vi "Recognize correct target fixed.vi"(9 "# rectangles":i32, 10 "Rectangles (Calibrated)":T2(array[cluster]), 11 "Image":T1) -> (3 "Image Out":T1)   [LabVIEW 2018]
uses:
  <vilib>/vision/Image Controls.llb/IMAQ Image.ctl
  Dashboard globals.vi
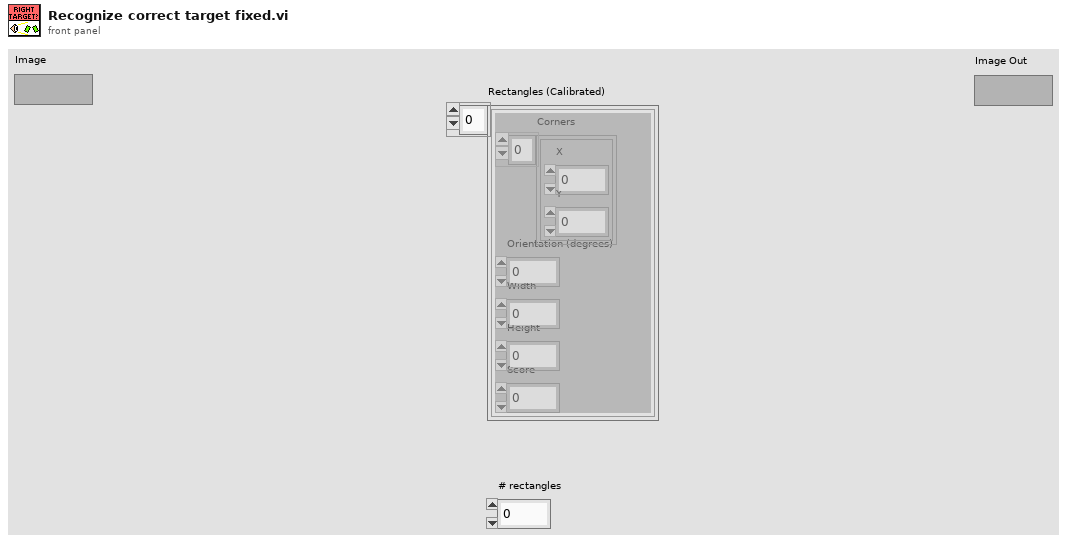
[diagram p1: front panel]
types:
  T1 = typedef "IMAQ Image.ctl" = refnum<image>
  T2 = cluster{"Corners":cluster{"X":sgl, "Y":sgl}[], "Orientation (degrees)":dbl, "Width":dbl, "Height":dbl, "Score":dbl}[]
  T3 = enum32{"Ship Left", "Ship Center", "Ship Right", "Rocket or Loading Station"}
  T4 = cluster{"Corners":cluster{"X":sgl, "Y":sgl}[], "Orientation (degrees)":dbl, "Width":dbl, "Height":dbl, "Score":dbl}
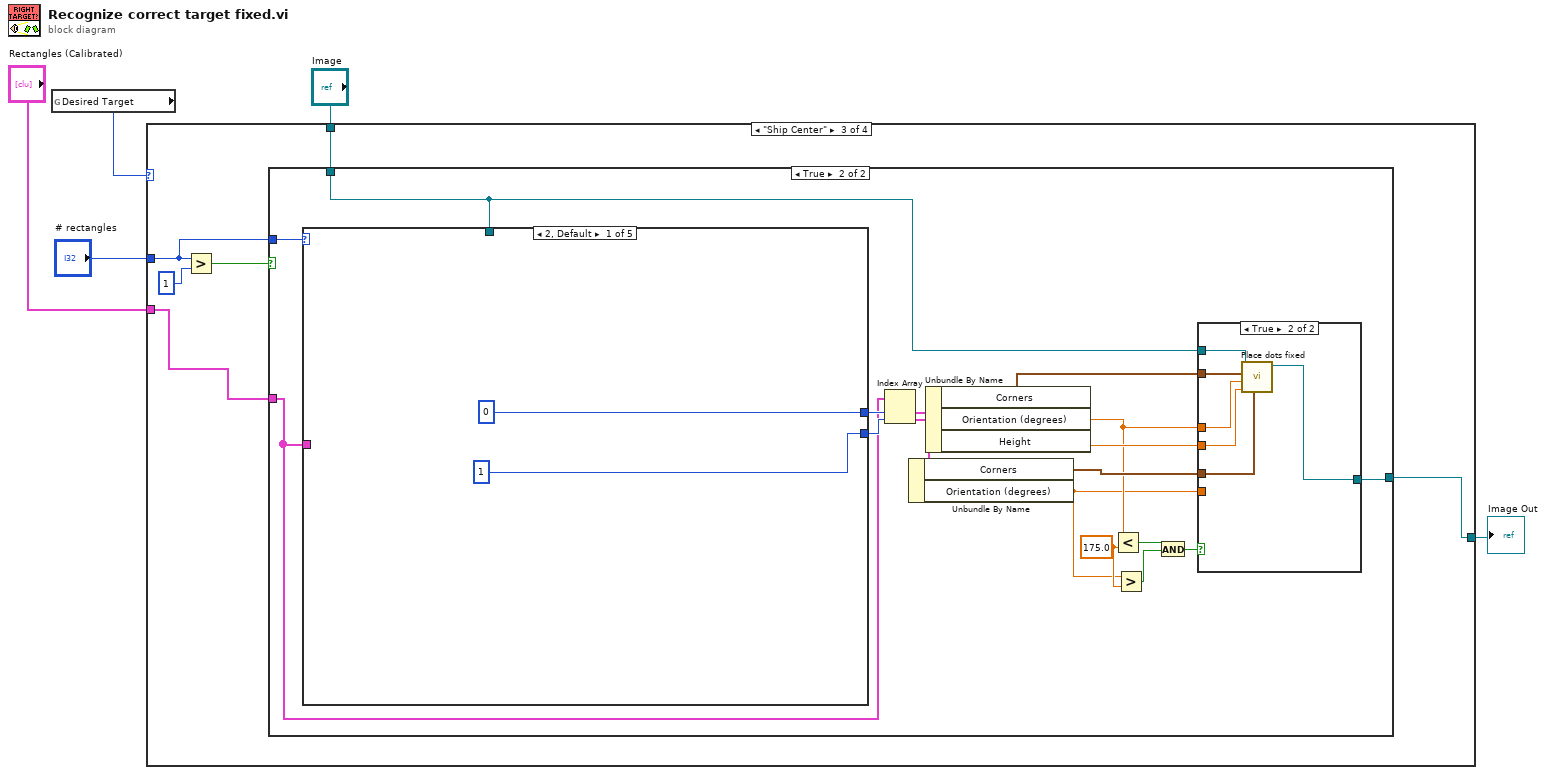
[diagram p0: block diagram]
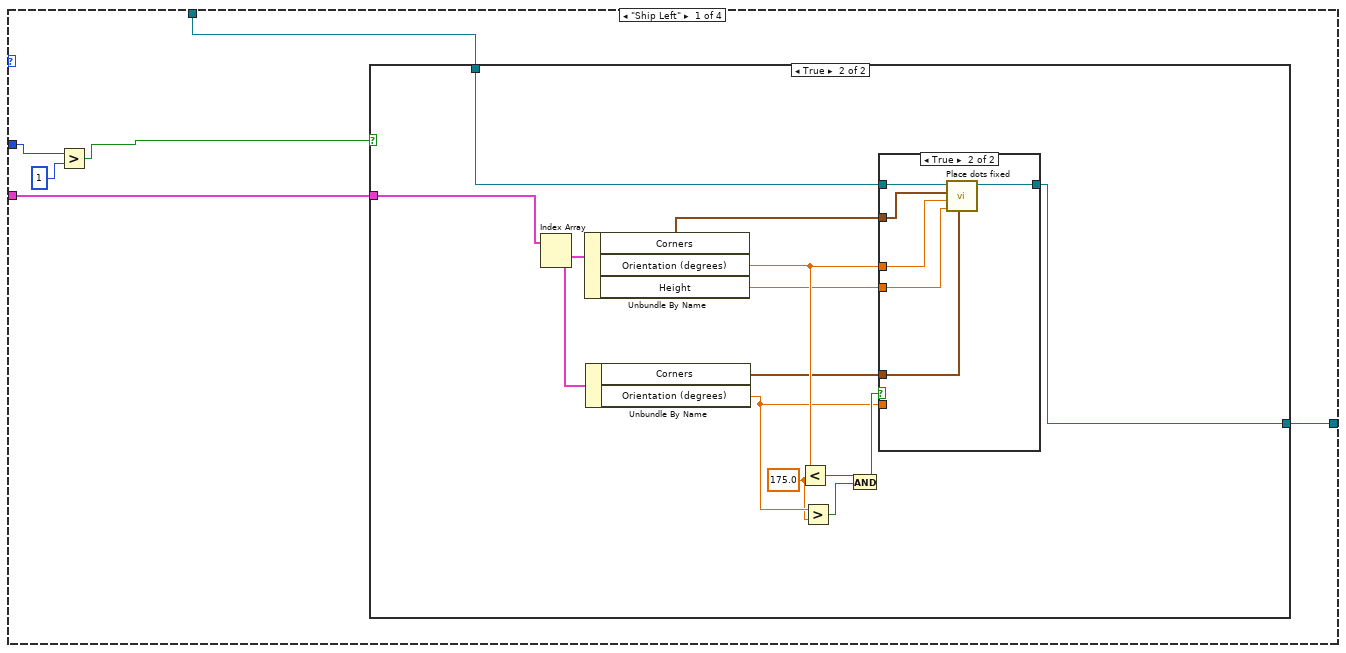
[diagram p2: hidden frame]
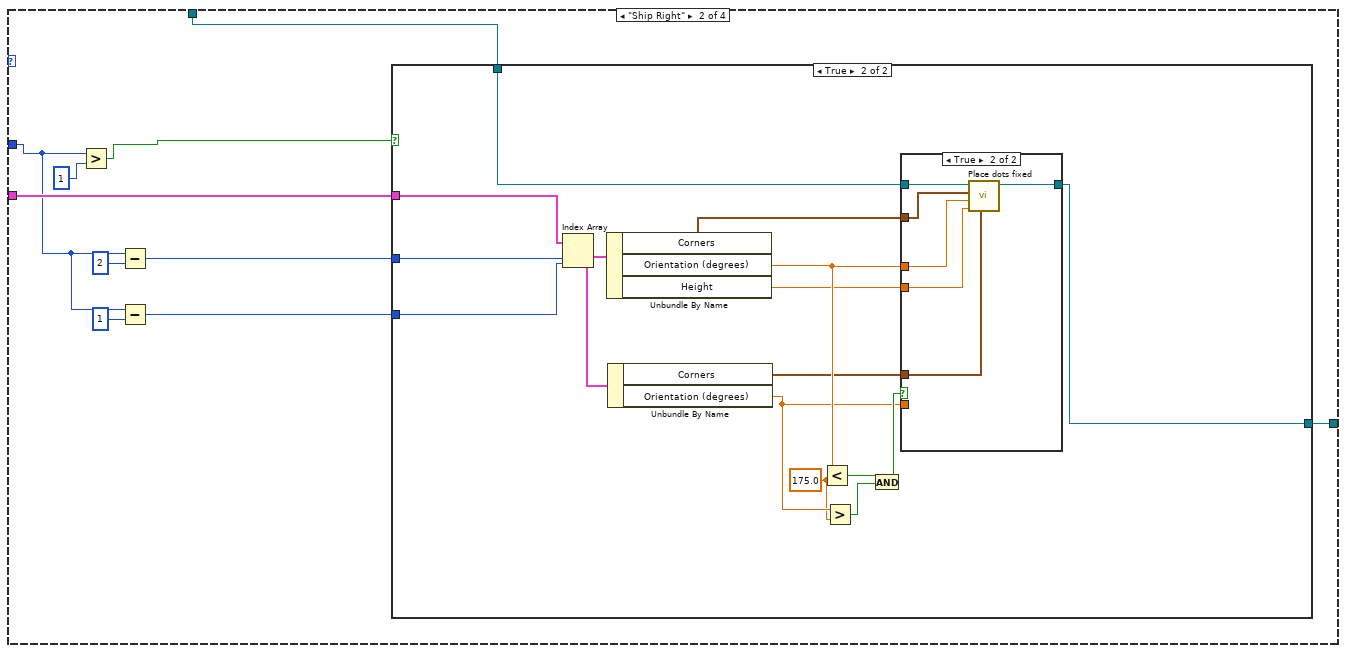
[diagram p5: hidden frame]
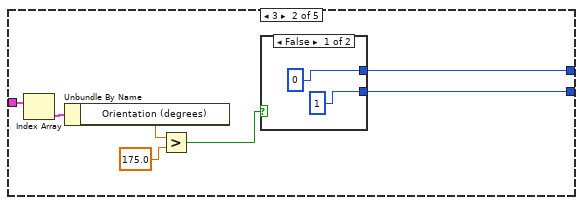
[diagram p9: hidden frame]
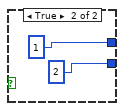
[diagram p10: hidden frame]
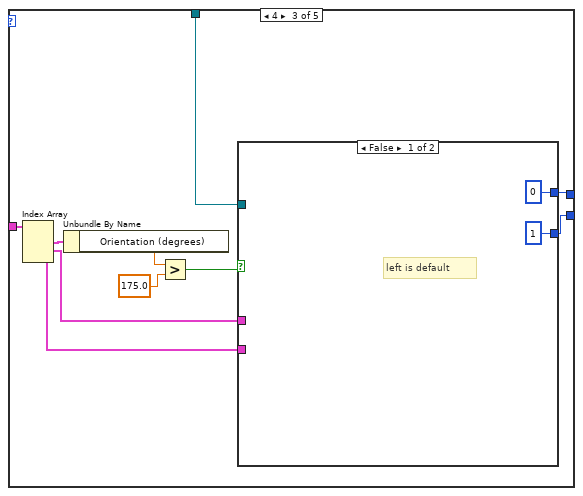
[diagram p11: hidden frame]
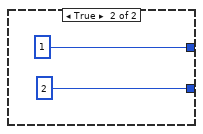
[diagram p12: hidden frame]
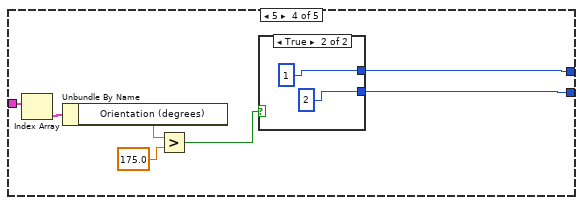
[diagram p13: hidden frame]
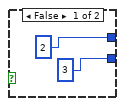
[diagram p14: hidden frame]
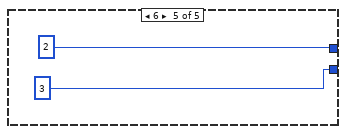
[diagram p15: hidden frame]
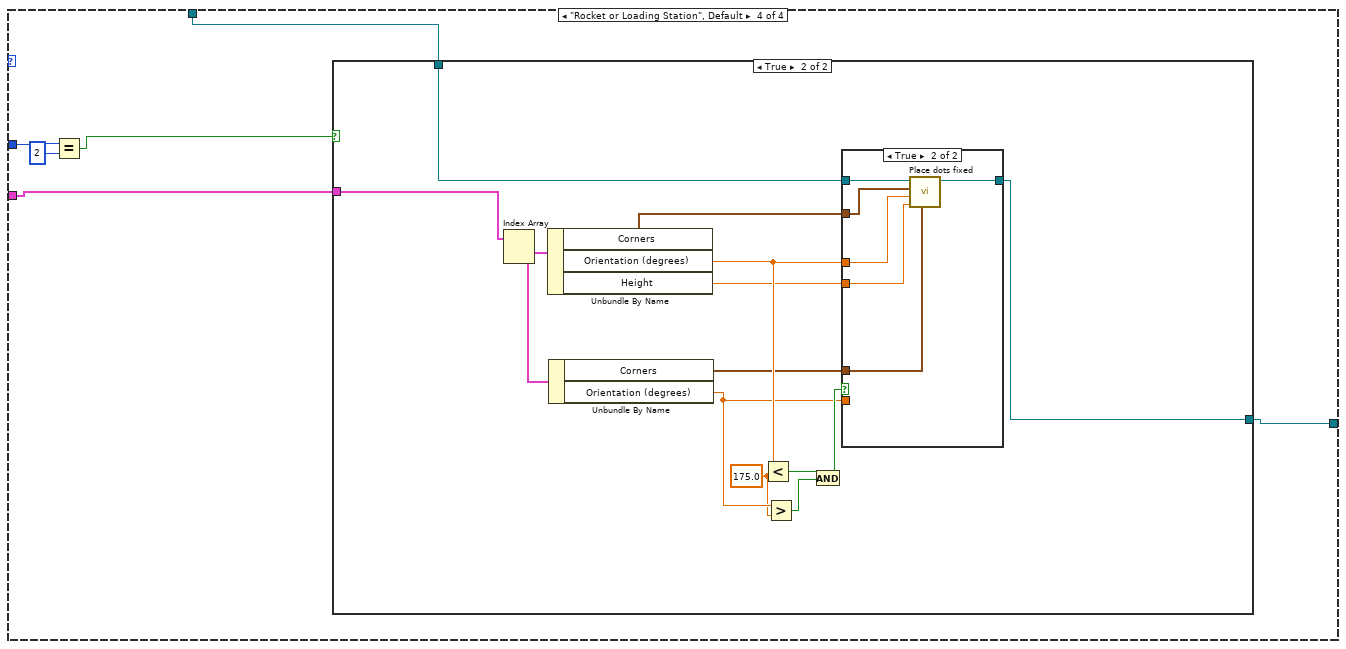
[diagram p17: hidden frame]
diagram:
  n1 = global read "Dashboard globals.vi" "Desired Target"() -> (w1:T3)
  n2 = case shown="\"Ship Center\"" w1 {
    tunnel: "Rectangles (Calibrated)" -> [w7 w41 w69 w141]
    tunnel: "Image" -> [w8 w40 w70 w140]
    tunnel: [w6 w39 w71 w139] -> w4
    tunnel: "# rectangles" -> [w11 w38 w68 w144]
    frame "Ship Left" {
      n3 = Greater?(x=w11, y=1) -> (0:w9:bool)
      n4 = case shown="True" w9 {
        tunnel: w8 -> [w12 w16]
        tunnel: w7 -> [_ w15]
        tunnel: [w12 w14] -> w6
        frame False {
        }
        frame True {
          w17 = 175.0 ("y")
          n5 = Index Array(array=w15) -> (element #1=w26:T4, element #2=w25:T4)  [unwired: 2 in]
          n6 = Unbundle By Name(w26) -> ("Corners"=w24:cluster{"X":sgl, "Y":sgl}[], "Orientation (degrees)"=w20:dbl, "Height"=w13:dbl)
          n7 = Unbundle By Name(w25) -> ("Corners"=w19:cluster{"X":sgl, "Y":sgl}[], "Orientation (degrees)"=w18:dbl)
          n8 = Less?(x=w20, y=w17) -> (x < y?=w23:bool)
          n9 = Greater?(x=w18, y=w17) -> (0:w22:bool)
          n10 = And(x=w23, y=w22) -> (x .and. y?=w21:bool)
          n11 = case shown="True" w21 {
            tunnel: w24 -> [_ w32]
            tunnel: w16 -> [w27 w33]
            tunnel: [w27 w31] -> w14
            tunnel: w20 -> [_ w30]
            tunnel: w19 -> [_ w28]
            tunnel: w18 -> [_ _]
            tunnel: w13 -> [_ w29]
            frame False {
            }
            frame True {
              n12 = call "Place dots fixed.vi"("Right Corner"=w28, "Left Height"=w29, "Left Orientation"=w30, "Left Corner"=w32, "Image IN"=w33) -> ("Image OUT"=w31:T1)  [unwired: 6 in]
            }
          }
        }
      }
    }
    frame "Ship Right" {
      n13 = Greater?(x=w38, y=1) -> (0:w42:bool)
      n14 = Subtract(x=w38, y=2) -> (x-y=w35:i32)
      n15 = Subtract(x=w38, y=1) -> (x-y=w34:i32)
      n16 = case shown="True" w42 {
        tunnel: w40 -> [w44 w50]
        tunnel: w41 -> [_ w49]
        tunnel: [w44 w48] -> w39
        tunnel: w35 -> [_ w46]
        tunnel: w34 -> [_ w45]
        frame False {
        }
        frame True {
          w51 = 175.0 ("y")
          n17 = Index Array(array=w49, index #1=w46, index #2=w45) -> (element #1=w60:T4, element #2=w59:T4)
          n18 = Unbundle By Name(w60) -> ("Corners"=w58:cluster{"X":sgl, "Y":sgl}[], "Orientation (degrees)"=w54:dbl, "Height"=w47:dbl)
          n19 = Unbundle By Name(w59) -> ("Corners"=w53:cluster{"X":sgl, "Y":sgl}[], "Orientation (degrees)"=w52:dbl)
          n20 = Less?(x=w54, y=w51) -> (x < y?=w57:bool)
          n21 = Greater?(x=w52, y=w51) -> (0:w56:bool)
          n22 = And(x=w57, y=w56) -> (x .and. y?=w55:bool)
          n23 = case shown="True" w55 {
            tunnel: w58 -> [_ w66]
            tunnel: w50 -> [w61 w67]
            tunnel: [w61 w65] -> w48
            tunnel: w54 -> [_ w64]
            tunnel: w53 -> [_ w62]
            tunnel: w52 -> [_ _]
            tunnel: w47 -> [_ w63]
            frame False {
            }
            frame True {
              n24 = call "Place dots fixed.vi"("Right Corner"=w62, "Left Height"=w63, "Left Orientation"=w64, "Left Corner"=w66, "Image IN"=w67) -> ("Image OUT"=w65:T1)  [unwired: 6 in]
            }
          }
        }
      }
    }
    frame "Ship Center" {
      n25 = Greater?(x=w68, y=1) -> (0:w72:bool)
      n26 = case shown="True" w72 {
        tunnel: [w74 w82] -> w71
        tunnel: w70 -> [w74 w77]
        tunnel: w69 -> [_ w78]
        tunnel: w68 -> [_ w81]
        frame False {
        }
        frame True {
          w83 = 175.0 ("y")
          n27 = case shown="2, Default" w81 {
            tunnel: [0 w95 w109 w120 2] -> w80
            tunnel: [1 w94 w108 w119 3] -> w79
            tunnel: w78 -> [_ w97 w111 w121 _]
            tunnel: w77 -> [_ _ w105 _ _]
            frame 2, Default {
            }
            frame 3 {
              n28 = Index Array(array=w97) -> (element=w99:T4)  [unwired: 1 in]
              n29 = Unbundle By Name(w99) -> ("Orientation (degrees)"=w100:dbl)
              n30 = Greater?(x=w100, y=175.0) -> (0:w96:bool)
              n31 = case shown="False" w96 {
                tunnel: [0 1] -> w95
                tunnel: [1 2] -> w94
                frame False {
                }
                frame True {
                }
              }
            }
            frame 4 {
              n32 = Index Array(array=w111) -> (element #1=w113:T4, element #2=w107:T4, element #3=w106:T4)  [unwired: 3 in]
              n33 = Unbundle By Name(w113) -> ("Orientation (degrees)"=w114:dbl)
              n34 = Greater?(x=w114, y=175.0) -> (0:w110:bool)
              n35 = case shown="False" w110 {
                tunnel: [0 1] -> w109
                tunnel: [1 2] -> w108
                tunnel: w107 -> [_ _]
                tunnel: w106 -> [_ _]
                tunnel: w105 -> [_ _]
                frame False {
                  # "left is default"
                }
                frame True {
                }
              }
            }
            frame 5 {
              n36 = Index Array(array=w121) -> (element=w124:T4)  [unwired: 1 in]
              n37 = Unbundle By Name(w124) -> ("Orientation (degrees)"=w123:dbl)
              n38 = Greater?(x=w123, y=175.0) -> (0:w125:bool)
              n39 = case shown="True" w125 {
                tunnel: [2 1] -> w120
                tunnel: [3 2] -> w119
                frame False {
                }
                frame True {
                }
              }
            }
            frame 6 {
            }
          }
          n40 = Index Array(array=w78, index #1=w80, index #2=w79) -> (element #1=w84:T4, element #2=w85:T4)
          n41 = Unbundle By Name(w85) -> ("Corners"=w87:cluster{"X":sgl, "Y":sgl}[], "Orientation (degrees)"=w75:dbl)
          n42 = Unbundle By Name(w84) -> ("Corners"=w86:cluster{"X":sgl, "Y":sgl}[], "Orientation (degrees)"=w76:dbl, "Height"=w91:dbl)
          n43 = Less?(x=w76, y=w83) -> (x < y?=w88:bool)
          n44 = Greater?(x=w75, y=w83) -> (0:w89:bool)
          n45 = And(x=w88, y=w89) -> (x .and. y?=w90:bool)
          n46 = case shown="True" w90 {
            tunnel: w86 -> [_ w137]
            tunnel: w87 -> [_ w133]
            tunnel: [w132 w136] -> w82
            tunnel: w91 -> [_ w135]
            tunnel: w77 -> [w132 w138]
            tunnel: w76 -> [_ w134]
            tunnel: w75 -> [_ _]
            frame False {
            }
            frame True {
              n47 = call "Place dots fixed.vi"("Right Corner"=w133, "Left Height"=w135, "Left Orientation"=w134, "Left Corner"=w137, "Image IN"=w138) -> ("Image OUT"=w136:T1)  [unwired: 6 in]
            }
          }
        }
      }
    }
    frame "Rocket or Loading Station", Default {
      n48 = Equal?(x=w144, y=2) -> (x = y?=w142:bool)
      n49 = case shown="True" w142 {
        tunnel: w140 -> [w145 w149]
        tunnel: w141 -> [_ w148]
        tunnel: [w145 w147] -> w139
        frame False {
        }
        frame True {
          w150 = 175.0 ("y")
          n50 = Index Array(array=w148) -> (element #1=w159:T4, element #2=w158:T4)  [unwired: 2 in]
          n51 = Unbundle By Name(w159) -> ("Corners"=w157:cluster{"X":sgl, "Y":sgl}[], "Orientation (degrees)"=w153:dbl, "Height"=w146:dbl)
          n52 = Unbundle By Name(w158) -> ("Corners"=w152:cluster{"X":sgl, "Y":sgl}[], "Orientation (degrees)"=w151:dbl)
          n53 = Less?(x=w153, y=w150) -> (x < y?=w156:bool)
          n54 = Greater?(x=w151, y=w150) -> (0:w155:bool)
          n55 = And(x=w156, y=w155) -> (x .and. y?=w154:bool)
          n56 = case shown="True" w154 {
            tunnel: w157 -> [_ w165]
            tunnel: w149 -> [w160 w166]
            tunnel: [w160 w164] -> w147
            tunnel: w153 -> [_ w163]
            tunnel: w152 -> [_ w161]
            tunnel: w151 -> [_ _]
            tunnel: w146 -> [_ w162]
            frame False {
            }
            frame True {
              n57 = call "Place dots fixed.vi"("Right Corner"=w161, "Left Height"=w162, "Left Orientation"=w163, "Left Corner"=w165, "Image IN"=w166) -> ("Image OUT"=w164:T1)  [unwired: 6 in]
            }
          }
        }
      }
    }
  }
  "Image Out" <- w4
